vi "tajriba_wahed.vi"() -> ()   [LabVIEW 2020]
panel:
  out "Sensor 1":bool
  in  "Banda":dbl(slide) scale=0.0..10.0
  in  "stop":bool
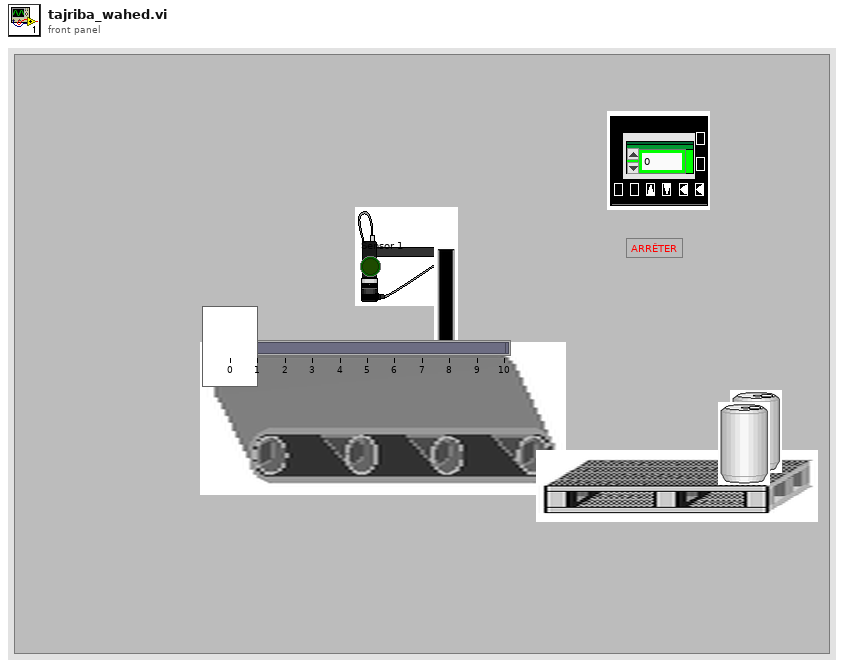
[diagram p1: front panel]
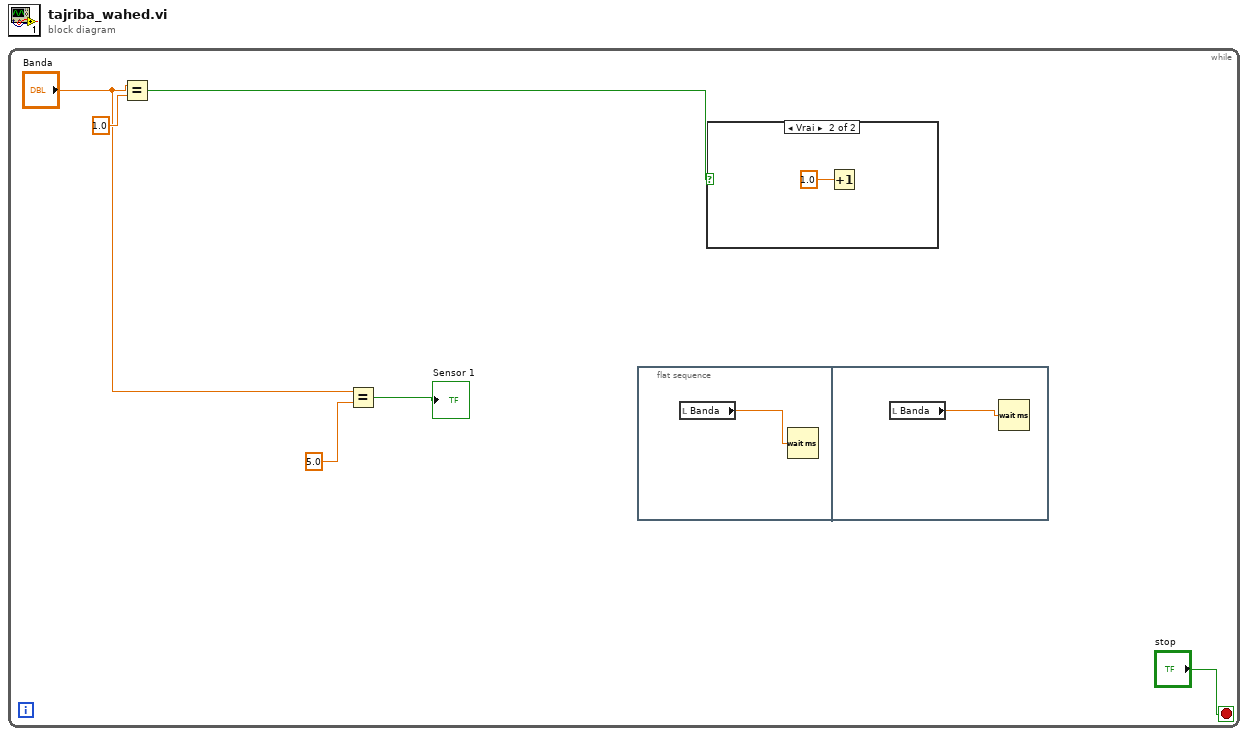
[diagram p0: block diagram]
diagram:
  n1 = while {
    stop <- "stop" stop-if-true
    n2 = Equal?(x="Banda", y=1.0) -> (x = y?=w4:bool)
    n3 = Equal?(x="Banda", y=5.0) -> (x = y?=→"Sensor 1":bool)
    n4 = flat-sequence {
      frame #0 {
        n5 = local read "Banda"() -> (w7:dbl)
        n6 = Wait (ms)(milliseconds to wait=w7) -> ()  [unwired: 1 out]
      }
      frame #1 {
        n7 = local read "Banda"() -> (w8:dbl)
        n8 = Wait (ms)(milliseconds to wait=w8) -> ()  [unwired: 1 out]
      }
    }
    n9 = case shown="Vrai" w4 {
      frame False {
      }
      frame True {
        n10 = Increment(x=1.0) -> ()  [unwired: 1 out]
      }
    }
  }
